vi "get_path_from_ver.vi"(0 "Version":string, 5 "Array":T1[](array[typedef])) -> (4 "Path":string)   [LabVIEW 2023, in "task_6.lvlib"]
doc: "Get the path of the given version."
uses:
  task_6.lvlib
  Controls/ver_path.ctl
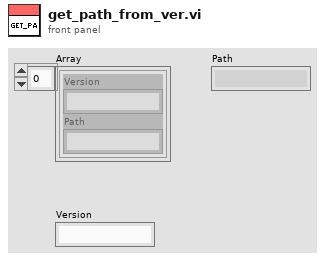
[diagram p1: front panel]
types:
  T1 = typedef "task_6.lvlib/ver_path.ctl" = cluster{"Version":string, "Path":string}
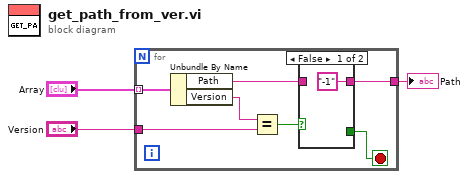
[diagram p0: block diagram]
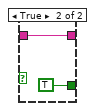
[diagram p2: hidden frame]
diagram:
  n1 = for {
    tunnel: "Array" -> [w10] mode=indexing
    tunnel: "Version" -> [w8]
    tunnel: [w4] -> w1
    stop <- w5 stop-if-true
    n2 = Unbundle By Name(w10) -> ("Path"=w6:string, "Version"=w9:string)
    n3 = Equal?(x=w9, y=w8) -> (x = y?=w7:bool)
    n4 = case shown="False" w7 {
      tunnel: w6 -> [_ w12]
      tunnel: [_ TRUE] -> w5
      tunnel: ["-1" ("Path") w12] -> w4
      frame False {
      }
      frame True {
      }
    }
  }
  "Path" <- w1
